vi "openeod V2.vi"(0 "file path":path, 5 "error in (no error)":errorcluster) -> (6 "Wave":i16[][](array[numeric]), 8 "nchar":u8[](array[numeric]), 9 "polarity":i8[](array[numeric]), 10 "nWavepoints":u32[](array[numeric]), 11 "userdata":sgl[][](array[numeric]), 12 "Numeric":i32, 13 "nbytes":i8[](array[numeric]), 14 "Byte Stream File out":refnum<file>, 15 "ADrange":sgl[](array[numeric]), 16 "eodtext":string[](array[string]), 17 "srate":u32[](array[numeric]), 18 "nbits":i8[](array[numeric]), 19 "error out":errorcluster)   [LabVIEW 2014]
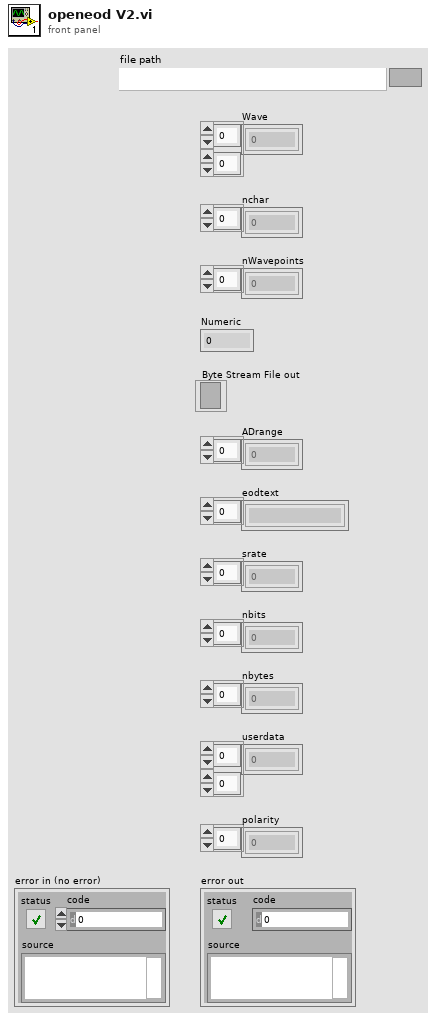
[diagram p1: front panel]
types:
  T1 = enum16{"open", "replace", "create", "open or create", "replace or create", "replace or create with confirmation"}
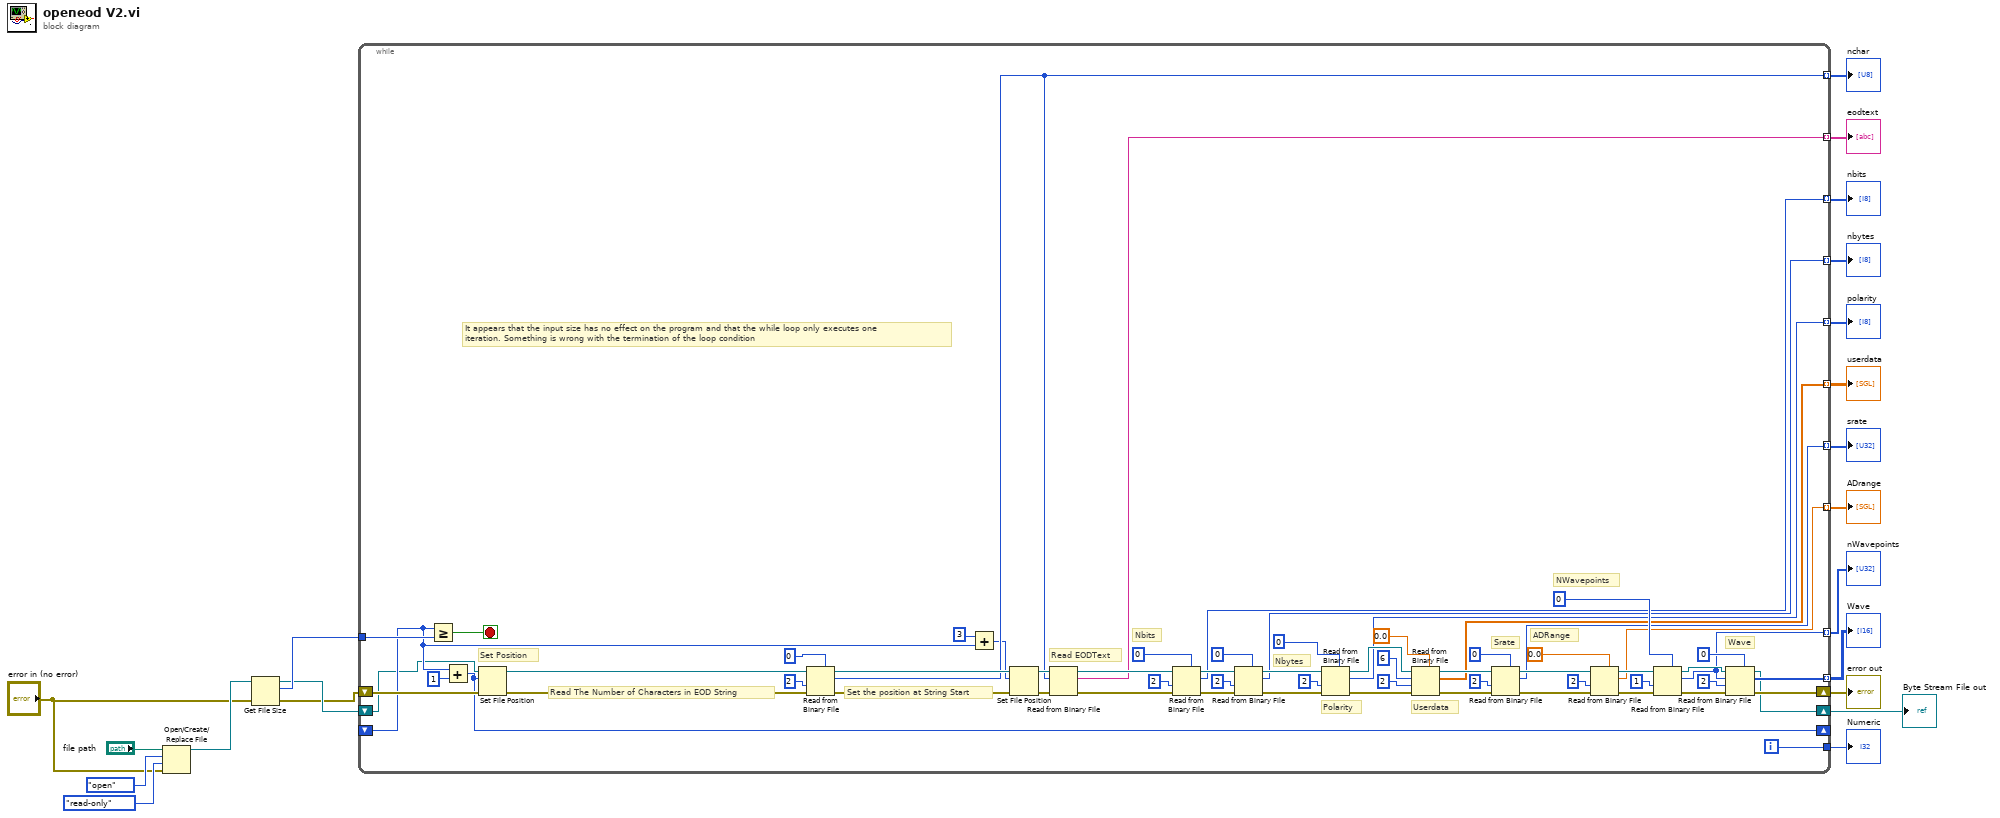
[diagram p0: block diagram]
diagram:
  n1 = Open/Create/Replace File(file path (use dialog)="file path", error in="error in (no error)", operation (0:open)=T1."open", access (0:read/write)=enum16{"read/write", "read-only", "write-only"}."read-only") -> (refnum out=w2:refnum<file>)  [unwired: 2 in, 2 out]
  n2 = Get File Size(file=w2, error in="error in (no error)") -> (refnum out=w6:refnum<file>, size (in bytes)=w7:i64)  [unwired: 1 out]
  n3 = while {
    tunnel: [w53] -> w8 mode=indexing
    tunnel: [w52] -> w9 mode=indexing
    tunnel: [w51] -> w10 mode=indexing
    tunnel: [w50] -> w11 mode=indexing
    tunnel: [w49] -> w12 mode=indexing
    tunnel: [w48] -> w13 mode=indexing
    tunnel: [w47] -> w14 mode=indexing
    tunnel: [w46] -> w15 mode=indexing
    tunnel: [w45] -> w17 mode=indexing
    tunnel: [w44] -> w16 mode=indexing
    shift-right: [w27] -> w19
    shift-left: w6 -> [w23]
    shift-right: [w31] -> w20
    shift-left: "error in (no error)" -> [w25]
    tunnel: w7 -> [w28]
    tunnel: [w26] -> w18
    shift-right: [w21] -> _
    shift-left: _ -> [w24]
    i -> [w26]
    stop <- w32 stop-if-true
    # "It appears that the input size has no effect on the program and that the while loop only executes one\niteration. Something is wrong with the termination of the loop condition"
    # "Wave"
    # "NWavepoints"
    # "ADRange"
    # "Srate"
    # "Userdata"
    # "Polarity"
    # "Nbytes"
    # "Nbits"
    # "Read EODText"
    # "Set the position at String Start"
    # "Read The Number of Characters in EOD String"
    # "Set Position"
    n4 = Greater Or Equal?(x=w24, y=w28) -> (x >= y?=w32:bool)
    n5 = Add(x=w24, y=1) -> (x+y=w21:i32)
    n6 = Set File Position(offset (in bytes) (0)=w21, refnum=w23, error in=w25) -> (refnum out=w82:refnum<file>, error out=w43:errorcluster)  [unwired: 1 in]
    n7 = Read from Binary File(5:u8 0, 8:w43, 9:2, 11:w82) -> (0:w42:errorcluster, 2:w53:u8, 3:w81:refnum<file>)  [unwired: 2 in, 1 out]
    n8 = Add(x=3, y=w24) -> (x+y=w22:i32)
    n9 = Set File Position(offset (in bytes) (0)=w22, refnum=w81, error in=w42) -> (refnum out=w80:refnum<file>, error out=w41:errorcluster)  [unwired: 1 in]
    n10 = Read from Binary File(8:w41, 10:w53, 11:w80) -> (0:w40:errorcluster, 2:w52:string, 3:w79:refnum<file>)  [unwired: 3 in, 1 out]
    n11 = Read from Binary File(5:i8 0, 8:w40, 9:2, 11:w79) -> (0:w39:errorcluster, 2:w51:i8, 3:w55:refnum<file>)  [unwired: 2 in, 1 out]
    n12 = Read from Binary File(5:i8 0, 8:w39, 9:2, 11:w55) -> (0:w38:errorcluster, 2:w50:i8, 3:w56:refnum<file>)  [unwired: 2 in, 1 out]
    n13 = Read from Binary File(5:i8 0, 8:w38, 9:2, 11:w56) -> (0:w37:errorcluster, 2:w49:i8, 3:w54:refnum<file>)  [unwired: 2 in, 1 out]
    n14 = Read from Binary File(5:sgl 0.0, 8:w37, 9:2, 10:6, 11:w54) -> (0:w36:errorcluster, 2:w48:sgl[], 3:w76:refnum<file>)  [unwired: 1 in, 1 out]
    n15 = Read from Binary File(5:u32 0, 8:w36, 9:2, 11:w76) -> (0:w35:errorcluster, 2:w47:u32, 3:w68:refnum<file>)  [unwired: 2 in, 1 out]
    n16 = Read from Binary File(5:sgl 0.0, 8:w35, 9:2, 11:w68) -> (0:w34:errorcluster, 2:w46:sgl, 3:w62:refnum<file>)  [unwired: 2 in, 1 out]
    n17 = Read from Binary File(5:u32 0, 8:w34, 9:1, 11:w62) -> (0:w33:errorcluster, 2:w44:u32, 3:w63:refnum<file>)  [unwired: 2 in, 1 out]
    n18 = Read from Binary File(5:i16 0, 8:w33, 9:2, 10:w44, 11:w63) -> (0:w31:errorcluster, 2:w45:i16[], 3:w27:refnum<file>)  [unwired: 1 in, 1 out]
  }
  "error out" <- w20
  "Byte Stream File out" <- w19
  "Numeric" <- w18
  "Wave" <- w17
  "nWavepoints" <- w16
  "ADrange" <- w15
  "srate" <- w14
  "userdata" <- w13
  "polarity" <- w12
  "nbytes" <- w11
  "nbits" <- w10
  "eodtext" <- w9
  "nchar" <- w8
